vi "Wrapper.vi"(0 "Send CRD Data in":refnum<class "Send CRD Data.lvclass">, 1 "Actor in":refnum<class "Actor.lvclass">, 5 "error in (no error)":errorcluster) -> (14 "Controller out":refnum<class "Controller.lvclass">, 19 "error out":errorcluster)   [LabVIEW 2014, in "Send CRD Data.lvclass"]
uses:
  Send CRD Data.lvclass
  Controller/Controller.lvclass
  reusable/CRDS/Data/Main/CRDS Data.lvclass
  Data/xData.lvclass
  <vilib>/ActorFramework/Actor/Actor.lvclass
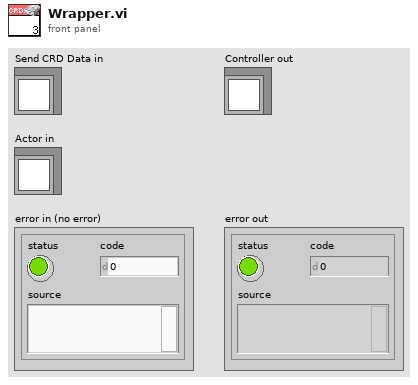
[diagram p1: front panel]
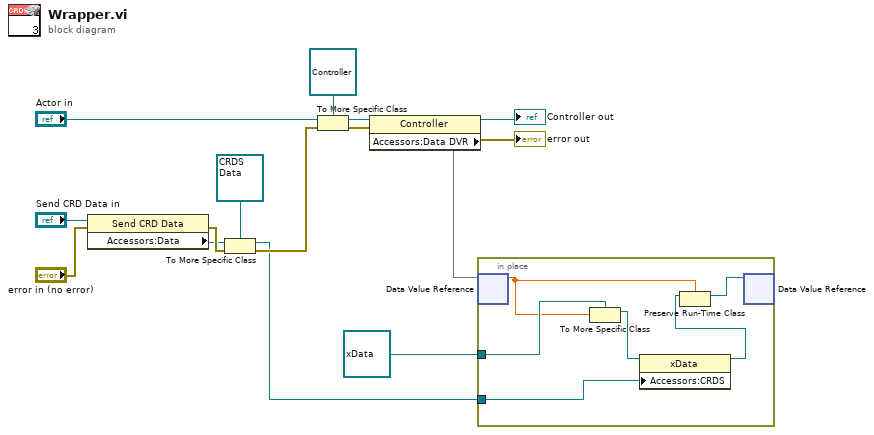
[diagram p0: block diagram]
diagram:
  n1 = property class="Send CRD Data"(reference="Send CRD Data in", error in="error in (no error)") -> (error out=w12:errorcluster, "Accessors:Data"=w9:refnum<class "Data.lvclass">)  [unwired: 1 out]
  n2 = To More Specific Class(target class=refnum<class "CRDS Data.lvclass"> refnum ("CRDS"), reference=w9, error in=w12) -> (specific class reference=w1:refnum<class "CRDS Data.lvclass">, error out=w11:errorcluster)
  n3 = To More Specific Class(target class=refnum<class "Controller.lvclass"> refnum ("Controller.lvlib:Controller"), reference="Actor in", error in=w11) -> (specific class reference=w8:refnum<class "Controller.lvclass">, error out=w13:errorcluster)
  n4 = property class="Controller"(reference=w8, error in=w13) -> (reference out=→"Controller out":refnum<class "Controller.lvclass">, error out=→"error out":errorcluster, "Accessors:Data DVR"=w3)
  n5 = in-place {
    in-place-border: refnum<class "xData.lvclass"> refnum ("xData.lvclass") -> [w20]
    in-place-border: w1 -> [w21]
    n6 = in-place-dvr #1(w3) -> (w17:dbl)  [unwired: 1 out]
    n7 = To More Specific Class(target class=w20, reference=w17) -> (specific class reference=w19:refnum<class "xData.lvclass">)  [unwired: 1 in, 1 out]
    n8 = property class="xData"(reference=w19, "Accessors:CRDS"=w21) -> (reference out=w18:refnum<class "xData.lvclass">)  [unwired: 1 in, 1 out]
    n9 = Preserve Run-Time Class(object in=w18, 2:w17) -> (object out=w16:refnum<class "Data.lvclass">)  [unwired: 1 in, 1 out]
    n10 = in-place-dvr #1(w16) -> ()  [unwired: 2 out]
  }
